vi "Mask Write Holding Register.vi"(4 "OR mask":u16, 6 "AND mask":u16, 8 "error in (no error)":errorcluster, 10 "address":u16, 11 "Modbus slave in":refnum<class "Modbus Slave.lvclass">) -> (0 "error out":errorcluster, 3 "Modbus slave out":refnum<class "Modbus Slave.lvclass">)   [LabVIEW 2020, in "Modbus Slave.lvclass"]
doc: "Writes values to one or more bits of a holding register."
uses:
  <vilib>/Modbus/slave/Modbus Slave.lvclass
  <vilib>/Modbus/slave/Modbus Slave.lvclass/Modbus Slave.ctl
  <vilib>/Modbus/subvis/Data and Functions/Device Data Model/Device Data Model.lvclass
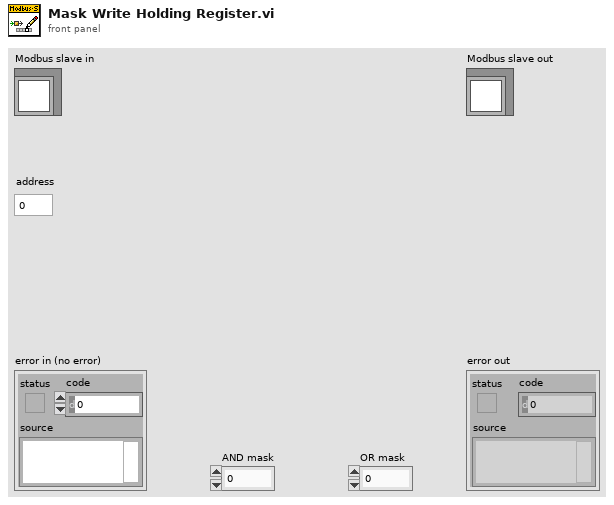
[diagram p1: front panel]
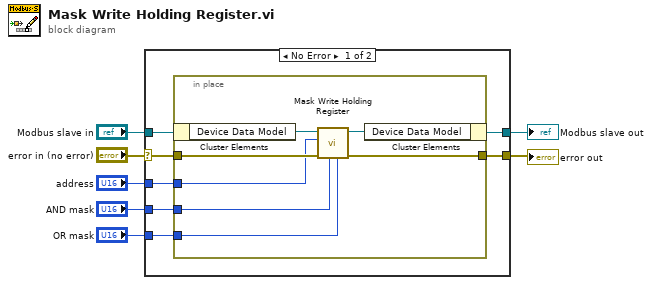
[diagram p0: block diagram]
diagram:
  n1 = case shown="No Error" "error in (no error)" {
    selector: "error in (no error)" -> [w12 w23]
    tunnel: [w13 w23] -> w6
    tunnel: "Modbus slave in" -> [w14 w22]
    tunnel: [w11 w22] -> w7
    tunnel: "address" -> [w10 _]
    tunnel: "AND mask" -> [w9 _]
    tunnel: "OR mask" -> [w8 _]
    frame No Error {
      n2 = in-place {
        in-place-border: [w20] -> w13
        in-place-border: w12 -> [w21]
        in-place-border: w10 -> [w17]
        in-place-border: w9 -> [w16]
        in-place-border: w8 -> [w15]
        n3 = in-place-cluster #1(w14) -> ("Device Data Model"=w19:refnum<class "Device Data Model.lvclass">)
        n4 = call-dynamic "Mask Write Holding Register.vi"("OR mask"=w15, "AND mask"=w16, "error in (no error)"=w21, "address"=w17, "device data model in"=w19) -> ("error out"=w20:errorcluster, "device data model out"=w18:refnum<class "Device Data Model.lvclass">)  [unwired: 5 in]
        n5 = in-place-cluster #1("Device Data Model"=w18) -> (w11:refnum<class "Modbus Slave.lvclass">)
      }
    }
    frame Error {
    }
  }
  "error out" <- w6
  "Modbus slave out" <- w7
